vi "Start.vi"(8 "error in (no error)":errorcluster, 10 "Params":variant, 11 "CorrFactor in":refnum<class "CorrFactor.lvclass">) -> (0 "error out":errorcluster, 3 "CorrFactor out":refnum<class "CorrFactor.lvclass">)   [LabVIEW 2018, in "AnalysisPlugins.lvlib" / "CorrFactor.lvclass"]
uses:
  CorrFactor.lvclass
  CorrFactor.lvclass/CorrFactor.ctl
  Accessors/Write 3458_Initialized.vi
  Accessors/Read 3458_Config.vi
  Accessors/Read 3458_Initialized.vi
  FitterBaseClass/FitterBase.lvclass
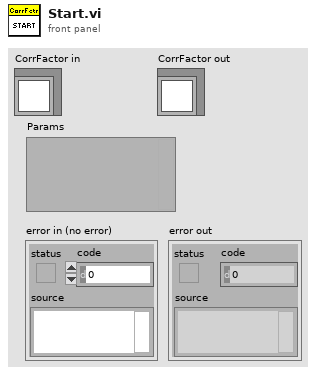
[diagram p1: front panel]
types:
  T1 = typedef "AnalysisPlugins.lvlib/CorrFactor.lvclass/clAnalysisConfig.ctl" = cluster{"HP 3458 address":string, "Amplitude":dbl, "3458  Params:":T2}
  T2 = typedef "AnalysisPlugins.lvlib/CorrFactor.lvclass/3458 Params.ctl" = cluster{"Record Size":i32, "Input Freq (Hz)":dbl, "# Cycles (Desired)":dbl, "Sampling Mode:":u16, "# of Record Avgs./Meas.":i32, "Trigger Mode":u16, "Trig. Level (%)":dbl, "# of Meas. Runs":i32, "Trigger Slope":u16}
  T3 = cluster{"Vin(s) (Vrms)":dbl[], "Vin phase(s) (deg)":dbl[], "Vin Freq. (Hz)":dbl}
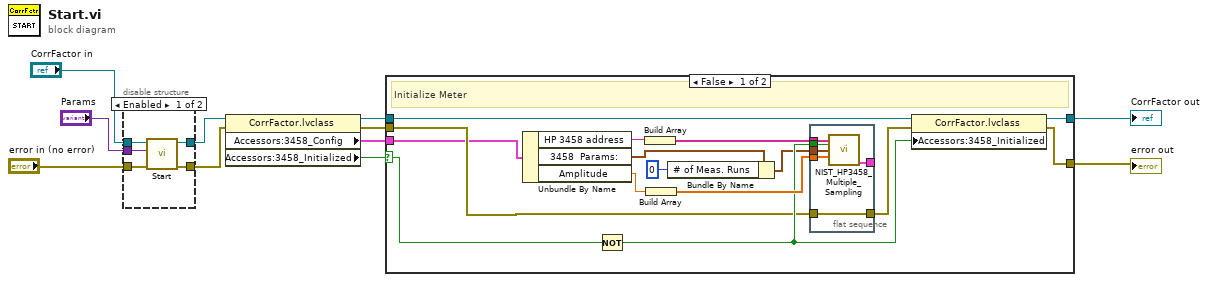
[diagram p0: block diagram]
diagram:
  n1 = disable-structure shown="Enabled" {
    disable-tunnel: [w16 w18] -> w11
    disable-tunnel: "error in (no error)" -> [w15 w17]
    disable-tunnel: "Params" -> [w14 _]
    disable-tunnel: "CorrFactor in" -> [w13 w18]
    disable-tunnel: [w12 w17] -> w7
    frame Enabled {
      n2 = call-parent "Start.vi"("error in (no error)"=w15, "Params"=w14, "FitterBase in"=w13) -> ("error out"=w12:errorcluster, "FitterBase out"=w16:refnum<class "CorrFactor.lvclass">)  [unwired: 7 in]
    }
    frame Disabled {
    }
  }
  n3 = property class="CorrFactor.lvclass"(reference=w11, error in=w7) -> (reference out=w2:refnum<class "CorrFactor.lvclass">, error out=w5:errorcluster, "Accessors:3458_Config"=w6:T1, "Accessors:3458_Initialized"=w3:bool)
  n4 = case shown="False" w3 {
    selector: w3 -> [w28 _]
    tunnel: w6 -> [w19 _]
    tunnel: w5 -> [w20 w40]
    tunnel: [w21 w40] -> w4
    tunnel: w2 -> [w29 w41]
    tunnel: [w26 w41] -> w1
    frame False {
      # "Initialize Meter"
      n5 = Unbundle By Name(w19) -> ("HP 3458 address"=w33:string, "3458  Params:"=w25:T2, "Amplitude"=w32:dbl)
      n6 = Not(x=w28) -> (.not. x?=w27:bool)
      n7 = Build Array(w33) -> (w31:string[])
      n8 = Build Array(w32) -> (w30:dbl[])
      n9 = Bundle By Name(cluster=w25, "# of Meas. Runs"=0) -> (w23:T2)
      n10 = flat-sequence {
        tunnel: w31 -> [w39]
        tunnel: w30 -> [w38]
        tunnel: w27 -> [w37]
        tunnel: w23 -> [w36]
        tunnel: [w35] -> w22
        tunnel: w20 -> [w35]
        tunnel: [w34] -> _
        frame #0 {
          n11 = call "NIST_HP3458_Multiple_Sampling.vi"("HP3458 Address(s):"=w39, "Initialize Meters:"=w37, "Input Sampling Parameters:"=w36, "HP3458 Input Voltage(s) (Vrms):"=w38) -> ("Averages"=w34:T3)  [unwired: 8 in, 3 out]
        }
      }
      n12 = property class="CorrFactor.lvclass"(reference=w29, error in=w22, "Accessors:3458_Initialized"=w27) -> (reference out=w26:refnum<class "CorrFactor.lvclass">, error out=w21:errorcluster)
    }
    frame True {
      # "Meter already initialized"
    }
  }
  "error out" <- w4
  "CorrFactor out" <- w1
